vi "Simple Read.vi"(4 "Class":refnum<class "Abs_U64 Integer 1D.lvclass">) -> (1 "Value":T1)   [LabVIEW 2021, in "Abs_U64 Integer 1D.lvclass"]
uses:
  Abs_U64 Integer 1D.lvclass
  Support/Type.ctl
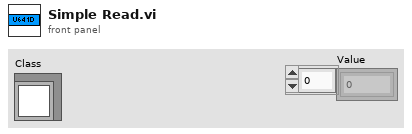
[diagram p1: front panel]
types:
  T1 = typedef "Abs_U64 Integer 1D.lvclass/Type.ctl" = u64[]
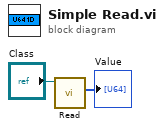
[diagram p0: block diagram]
diagram:
  n1 = call-dynamic "Read.vi"("Double Float.lvclass_340760 in"="Class") -> ("Value"=→"Value":T1)  [unwired: 8 in, 2 out]
